vi "Read Enabled_.vi"(8 "error in (no error)":errorcluster, 11 "Lesker Pressure in":refnum<class "Lesker Pressure.lvclass">) -> (0 "error out":errorcluster, 2 "Enabled?":bool[](array[boolean]), 3 "Lesker Pressure out":refnum<class "Lesker Pressure.lvclass">)   [LabVIEW 2024, in "Lesker Pressure.lvclass"]
uses:
  Lesker Pressure.lvclass
  Lesker Pressure.lvclass/Lesker Pressure.ctl
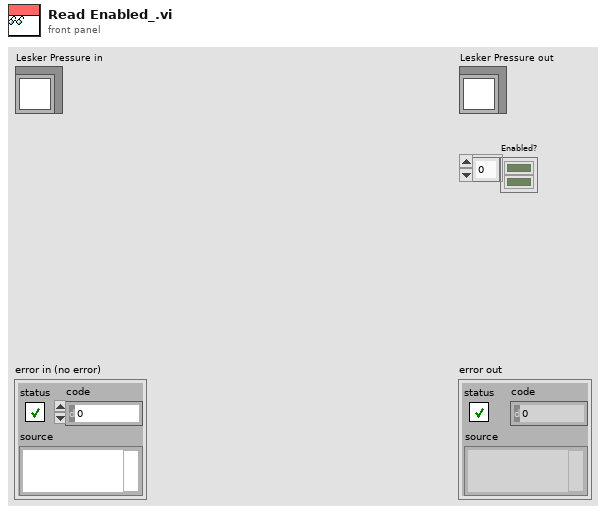
[diagram p1: front panel]
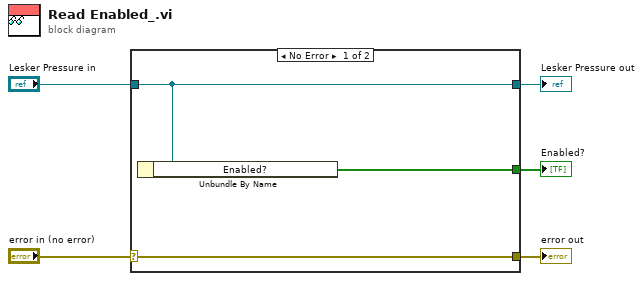
[diagram p0: block diagram]
diagram:
  n1 = case shown="No Error" "error in (no error)" {
    selector: "error in (no error)" -> [w8 w9]
    tunnel: [w8 w9] -> w4
    tunnel: [w7 w10] -> w2
    tunnel: "Lesker Pressure in" -> [w7 w10]
    tunnel: [w6 _] -> w1
    frame No Error {
      n2 = Unbundle By Name(w7) -> ("Enabled?"=w6:bool[])
    }
    frame Error {
    }
  }
  "error out" <- w4
  "Lesker Pressure out" <- w2
  "Enabled?" <- w1
